vi "Contour Finding Test.vi"() -> ()   [LabVIEW 2011]
uses:
  <vilib>/vision/Analysis.llb/IMAQ ExtractCurvesCurve.ctl
  <vilib>/vision/Pattern Matching.llb/IMAQ Curve Parameters.ctl
  <vilib>/vision/NI_Vision_Development_Module.lvlib
panel:
  in  "Curve Parameters":T1={"Extraction Mode"=0, "Edge Threshold"=75, "Edge Filter Size"=1, "Min Length"=25, "Row Search Step Size"=15, "Col Search Step Size"=15, "Max Endpoint Gap"=10, "Closed"=FALSE, "Subpixel"=FALSE} {"Extraction Mode" items=["Normal", "Uniform Regions"]; "Edge Filter Size" items=["Fine", "Normal", "Contour Tracing"]; "Max Endpoint Gap" min=0; "Col Search Step Size" min=1 max=255 step=1; "Row Search Step Size" min=1 max=255 step=1; "Min Length" min=0; "Edge Threshold" min=1 max=350 step=1}
  out "Original image":T2(plugin-control)
  out "Curves":T3[](array[typedef]) {"Points"."Y" format="%.2f"; "Points"."X" format="%.2f"}
  out "Thresholded":T2(plugin-control)
  in  "Range":cluster{"Lower value":sgl, "Upper value":sgl}={"Lower value"=3000.0, "Upper value"=32768.0} {"Upper value" format="%.2f"; "Lower value" format="%.2f"}
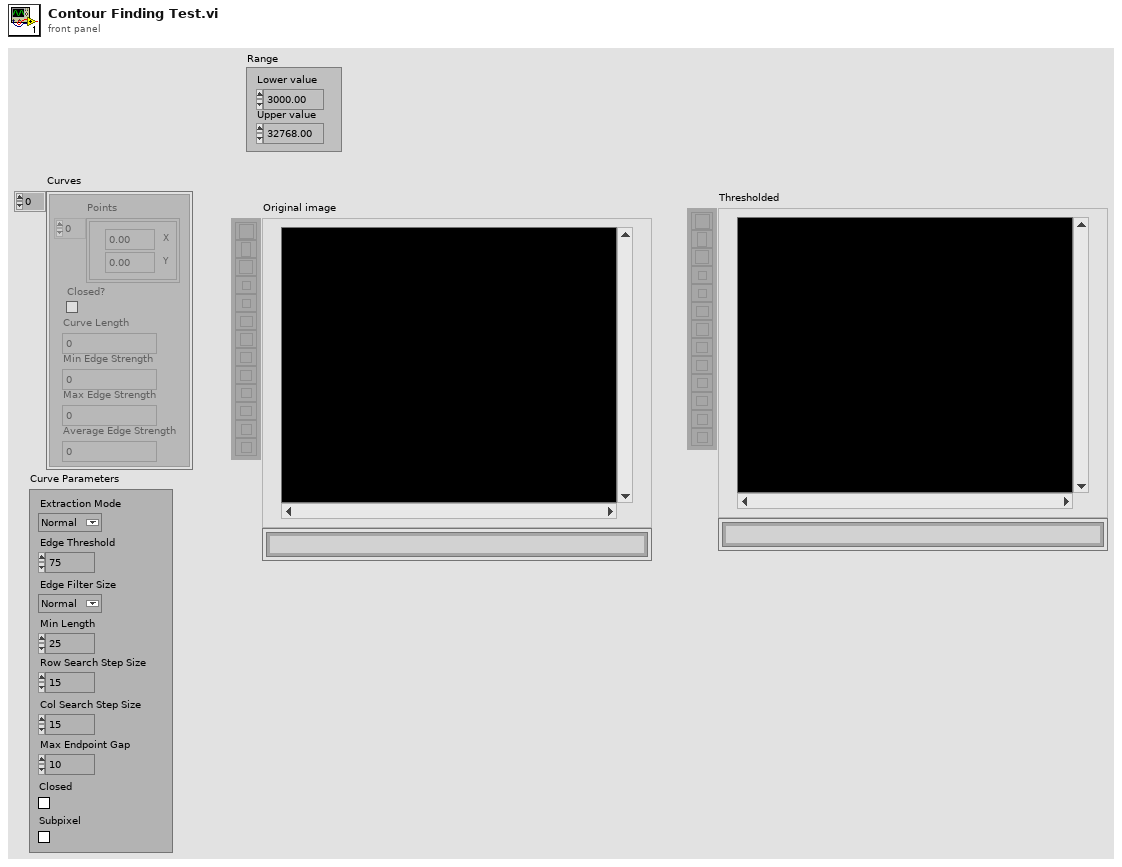
[diagram p1: front panel]
types:
  T1 = typedef "IMAQ Curve Parameters.ctl" = cluster{"Extraction Mode":u32, "Edge Threshold":i32, "Edge Filter Size":u32, "Min Length":i32, "Row Search Step Size":i32, "Col Search Step Size":i32, "Max Endpoint Gap":i32, "Closed":bool, "Subpixel":bool}
  T2 = typedef "IMAQ Image.ctl" = refnum<image>
  T3 = typedef "IMAQ ExtractCurvesCurve.ctl" = cluster{"Points":cluster{"X":dbl, "Y":dbl}[], "Closed?":bool, "Curve Length":dbl, "Min Edge Strength":dbl, "Max Edge Strength":dbl, "Average Edge Strength":dbl}
  T4 = typedef "Image Type" = u32
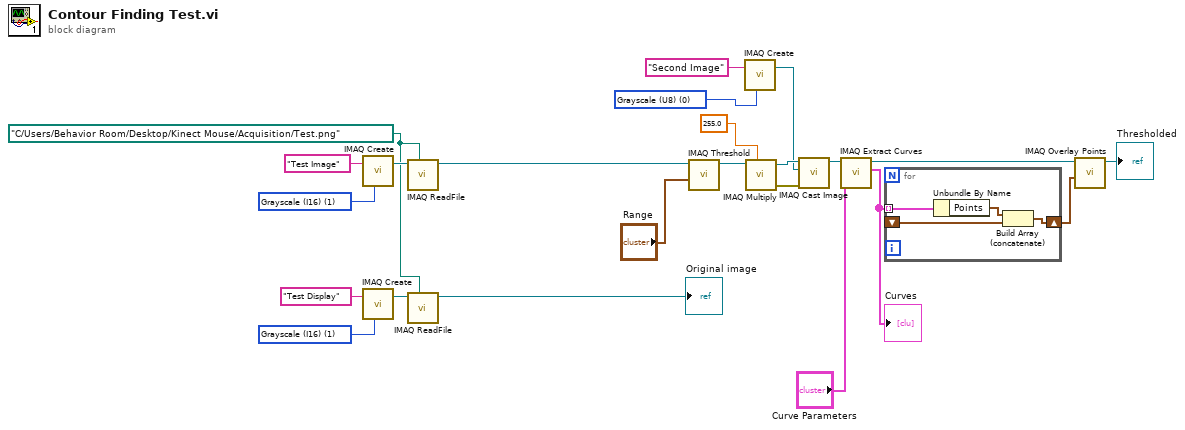
[diagram p0: block diagram]
diagram:
  w12 = T4 1 items=["Grayscale (U8)", "Grayscale (I16)", "Grayscale (SGL)", "Complex (CSG)", "RGB (U32)", "HSL (U32)", "RGB (U64)", "Grayscale (U16)"] ("Image Type")
  w15 = T4 0 items=["Grayscale (U8)", "Grayscale (I16)", "Grayscale (SGL)", "Complex (CSG)", "RGB (U32)", "HSL (U32)", "RGB (U64)", "Grayscale (U16)"] ("Image Type")
  w8 = path "C:/Users/Behavior Room/Desktop/Kinect Mouse/Acquisition/Test.png" ("File Path")
  w23 = T4 1 items=["Grayscale (U8)", "Grayscale (I16)", "Grayscale (SGL)", "Complex (CSG)", "RGB (U32)", "HSL (U32)", "RGB (U64)", "Grayscale (U16)"] ("Image Type")
  n1 = call "IMAQ Create"("Image Name"="Test Image", "Image Type"=w23) -> ("New Image"=w21:T2)  [unwired: 3 in, 1 out]
  n2 = call "IMAQ Create"("Image Name"="Test Display", "Image Type"=w12) -> ("New Image"=w10:T2)  [unwired: 3 in, 1 out]
  n3 = call "IMAQ ReadFile"("File Path"=w8, "Image"=w21) -> ("Image Out"=w13:T2)  [unwired: 5 in, 4 out]
  n4 = call "IMAQ ReadFile"("File Path"=w8, "Image"=w10) -> ("Image Out"=→"Original image":T2)  [unwired: 5 in, 4 out]
  n5 = call "IMAQ Threshold"("Range"="Range", "Image Src"=w13) -> ("Image Dst Out"=w19:T2)  [unwired: 8 in, 1 out]
  n6 = call "IMAQ Create"("Image Name"="Second Image", "Image Type"=w15) -> ("New Image"=w14:T2)  [unwired: 3 in, 1 out]
  n7 = call "IMAQ Multiply"("Image Src A"=w19, "Constant"=sgl 255.0) -> ("Image Dst Out"=w17:T2, "error out"=w18:errorcluster)  [unwired: 5 in]
  n8 = call "IMAQ Cast Image"("error in (no error)"=w18, "Image Dst"=w14, "Image Src"=w17) -> ("Image Dst Out"=w6:T2)  [unwired: 7 in, 1 out]
  n9 = call "IMAQ Extract Curves"("Curve Parameters"="Curve Parameters", "Image"=w6) -> ("Curves"=w2:T3[], "Image (dup)"=w5:T2)  [unwired: 7 in, 1 out]
  "Curves" <- w2
  n10 = for {
    tunnel: w2 -> [w27] mode=indexing
    shift-right: [w25] -> w3
    shift-left: _ -> [w24]
    n11 = Unbundle By Name(w27) -> ("Points"=w26:cluster{"X":dbl, "Y":dbl}[])
    n12 = Build Array (concatenate)(w26, w24) -> (w25:cluster{"X":dbl, "Y":dbl}[])
  }
  n13 = call "IMAQ Overlay Points"("Array of Points"=w3, "Image"=w5) -> ("Image Out"=→"Thresholded":T2)  [unwired: 8 in, 1 out]
